vi "RSZVB Set UI Signal Pin 21.vi"(8 "error in (no error)":errorcluster {"code" format="%.0x"}, 9 "Pin 21 (Off)":bool, 11 "VISA session":refnum<visa-resource-name>) -> (0 "error out":errorcluster {"code" format="%.0x"}, 3 "dup VISA session":refnum<visa-resource-name>)   [LabVIEW 2011]
doc: "This VI selects the digital signal that is routed to pin 21 of the Universal Interface connector.\n\nRemote-control command(s):\nCONTrol:HANDler[:EXTension]:RTRigger:STATe"
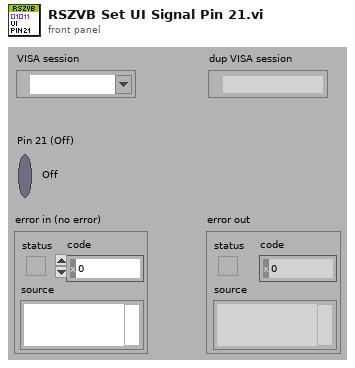
[diagram p1: front panel]
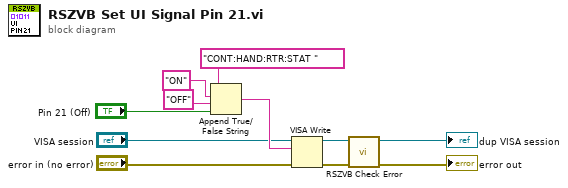
[diagram p0: block diagram]
diagram:
  n1 = Append True/False String(1:"Pin 21 (Off)", 2:"OFF", 3:"ON", 4:"CONT:HAND:RTR:STAT ") -> (0:w6:string)
  n2 = VISA Write(VISA resource name="VISA session", write buffer=w6, error in (no error)="error in (no error)") -> (VISA resource name out=w10:refnum<visa-resource-name>, error out=w11:errorcluster)  [unwired: 1 out]
  n3 = call "RSZVB Check Error.vi"("error in (no error)"=w11, "VISA session"=w10) -> ("error out"=→"error out":errorcluster, "dup VISA session"=→"dup VISA session":refnum<visa-resource-name>)  [unwired: 8 in]
